vi "liblinear_train_example.vi"(8 "error in (no error)":errorcluster) -> (0 "error out":errorcluster, 3 "Binary Confusion Matrix":T1)   [LabVIEW 2015]
uses:
  Tools/Controls/Binary_ConfusionMatrix.ctl
  Controls/liblinear_problem.ctl
  LibSVM Sparse/Wrapper API/Controls/svm_node.ctl
  Controls/liblinear_parameter.ctl
  Controls/liblinear_solver.ctl
  Tools/SubVIs/Sparse - Scale Nodes Linear.vi
  Tools/SubVIs/Liblinear - Split Problem.vi
  Tools/SubVIs/Liblinear - Scale Problem Linear.vi
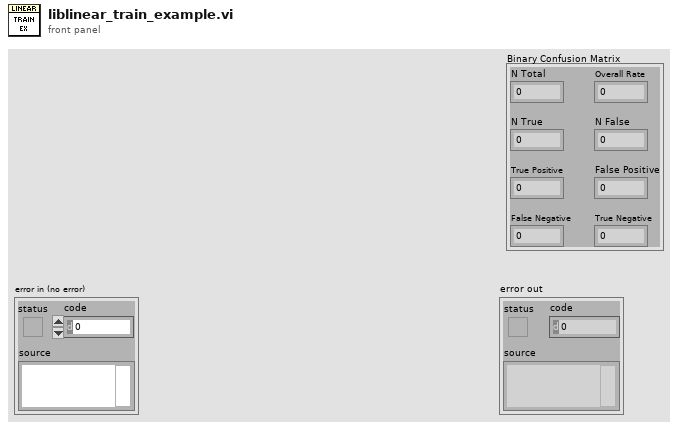
[diagram p1: front panel]
types:
  T1 = typedef "Binary_ConfusionMatrix.ctl" = cluster{"N Total":u32, "N True":u32, "N False":u32, "Overall Rate":dbl, "True Positive":dbl, "False Positive":dbl, "False Negative":dbl, "True Negative":dbl}
  T2 = typedef "liblinear_parameter.ctl" = cluster{"solver_type":T3, "eps":dbl, "C":dbl, "weight_label":i32[], "weight":dbl[], "p":dbl}
  T3 = typedef "liblinear_solver.ctl" = u32
  T4 = typedef "liblinear_problem.ctl" = cluster{"y":dbl[], "x":cluster{T5[]}[], "bias":dbl}
  T5 = typedef "svm_node.ctl" = cluster{"index":i32, "value":dbl}
  T6 = typedef "svm_problem.ctl" = cluster{"y":dbl[], "x":cluster{T5[]}[]}
  T7 = typedef "liblinear_model.ctl" = cluster{"liblinear_parameter":T2, "nr_class":i32, "nr_feature":i32, "w":dbl[], "label":i32[], "bias":dbl}
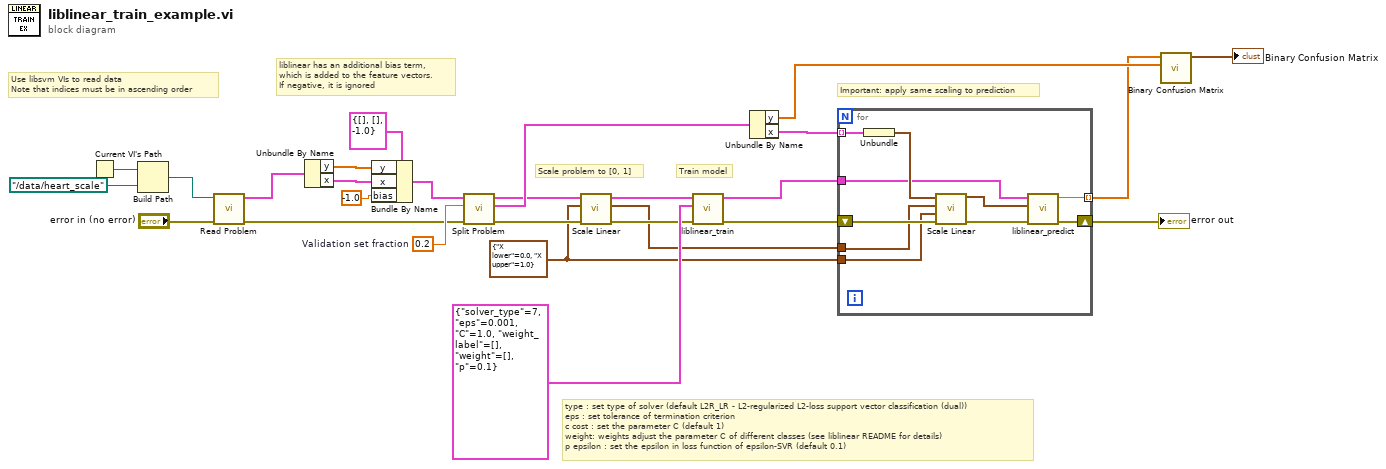
[diagram p0: block diagram]
diagram:
  w1 = cluster{"X lower":dbl, "X upper":dbl} {"X lower"=0.0, "X upper"=1.0} ("X Scaling limits")
  w18 = 0.2  # Validation set fraction
  # "Important: apply same scaling to prediction"
  # "Train model"
  # "Scale problem to [0, 1]"
  # "type : set type of solver (default L2R_LR - L2-regularized L2-loss support vector classification (dual))\neps : set tolerance of termination criterion\nc cost : set the parameter C (default 1)\nweight: weights adjust the parameter C of different classes (see liblinear README for details)\np epsilon : set the epsilon in loss function of epsilon-SVR (default 0.1)"
  # "liblinear has an additional bias term, \nwhich is added to the feature vectors.\nIf negative, it is ignored"
  # "Use libsvm VIs to read data\nNote that indices must be in ascending order"
  n1 = Current VI's Path() -> (path=w27:path)
  n2 = Build Path(base path=w27, name or relative path=path "../data/heart_scale" ("file path (use dialog)")) -> (appended path=w25:path)
  n3 = call "Read Problem.vi"("error in (no error)"="error in (no error)", "file path (use dialog)"=w25) -> ("error out"=w12:errorcluster, "svm_problem"=w13:T6)  [unwired: 8 in]
  n4 = Unbundle By Name(w13) -> ("y"=w2:dbl[], "x"=w23:cluster{T5[]}[])
  n5 = Bundle By Name(cluster=T4 {"y"=[], "x"=[], "bias"=-1.0} ("liblinear_problem"), "y"=w2, "x"=w23, "bias"=-1.0) -> (w19:T4)
  n6 = call-poly "Split Problem.vi"("error in (no error)"=w12, "Validation fraction"=w18, "liblinear_problem"=w19) -> ("error out"=w11:errorcluster, "Validation set"=w16:T4, "Training set"=w10:T4)  [unwired: 4 in, 2 out]
  n7 = call-poly "Scale Linear.vi"("error in (no error)"=w11, "X Scaling limits"=w1, "Problem"=w10) -> ("error out"=w9:errorcluster, "xmaxmin"=w6:cluster{"min":dbl, "max":dbl}[], "Scaled problem"=w8:T4)  [unwired: 6 in]
  n8 = call "liblinear_train.vi"("error in (no error)"=w9, "parameters"=T2 {"solver_type"=7, "eps"=0.001, "C"=1.0, "weight_label"=[], "weight"=[], "p"=0.1}, "problem"=w8) -> ("error out"=w14:errorcluster, "model"=w15:T7)  [unwired: 7 in]
  n9 = Unbundle By Name(w16) -> ("y"=w4:dbl[], "x"=w7:cluster{T5[]}[])
  n10 = for {
    tunnel: w15 -> [w32]
    shift-right: [w29] -> w5
    shift-left: w14 -> [w37]
    tunnel: w7 -> [w36] mode=indexing
    tunnel: w6 -> [w34]
    tunnel: w1 -> [w33]
    tunnel: [w28] -> w3 mode=indexing
    n11 = Unbundle(w36) -> (w35:T5[])
    n12 = call-poly "Scale Linear.vi"("error in (no error)"=w37, "Scaling limits"=w33, "xmaxmin"=w34, "x"=w35) -> ("error out"=w30:errorcluster, "x scaled"=w31:T5[])  [unwired: 6 in]
    n13 = call "liblinear_predict.vi"("error in (no error)"=w30, "x"=w31, "liblinear_model"=w32) -> ("error out"=w29:errorcluster, "predicted label"=w28:dbl)  [unwired: 7 in]
  }
  "error out" <- w5
  n14 = call "Binary Confusion Matrix.vi"("Actual Labels"=w4, "Predicted Labels"=w3) -> ("Binary Confusion Matrix"=→"Binary Confusion Matrix":T1)  [unwired: 8 in, 1 out]
